vi "Average tau0.vi"(4 "filter changed?":bool, 6 "filter":bool, 8 "error in":errorcluster, 9 "# of shots":i32, 10 "extParam":T1={"Tau"=nan, "Tau0cor"=nan, "ext"=nan, "extCorr"=nan, "stdevTau"=nan, "eTau"=nan, "taucorr"=nan, "Tau0"=nan, "max"=nan}, 11 "CRDS Cell in":refnum<class "CRDS Cell.lvclass">) -> (0 "error out":errorcluster, 3 "CRDS Cell out":refnum<class "CRDS Cell.lvclass">)   [LabVIEW 2014, in "CRDS Lib.lvlib" / "CRDS Cell.lvclass"]
doc: "Average taus recorded on filter to give a mean tau0. The values tau0 and tau0cor will be averaged over the number of times this vi is called or the value of <b># of shots</b>, whichever is smaller.\n\nOnly accessors can throw errors here."
uses:
  CRDS Cell.lvclass
  extParam Ctl.ctl
  CRDS Cell.lvclass/CRDS Cell.ctl
  Data/Cell/CRDS Cell Data.lvclass/CRDS Cell Data.ctl
  <vilib>/Analysis/baseanly.llb/Mean (DBL).vi
  Read Data.vi
  Data/Cell/Write extParam.vi
  Write Data.vi
  Write corr tau0.vi
  Write tau_0.vi
  Data/Cell/CRDS Cell Data.lvclass
  <vilib>/Analysis/NI_AALBase.lvlib
  CRDS Lib.lvlib
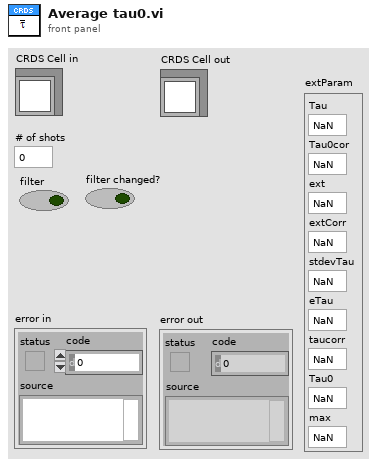
[diagram p1: front panel]
types:
  T1 = typedef "CRDS Lib.lvlib/extParam Ctl.ctl" = cluster{"Tau":sgl, "Tau0cor":sgl, "ext":sgl, "extCorr":sgl, "stdevTau":sgl, "eTau":sgl, "taucorr":sgl, "Tau0":sgl, "max":sgl}
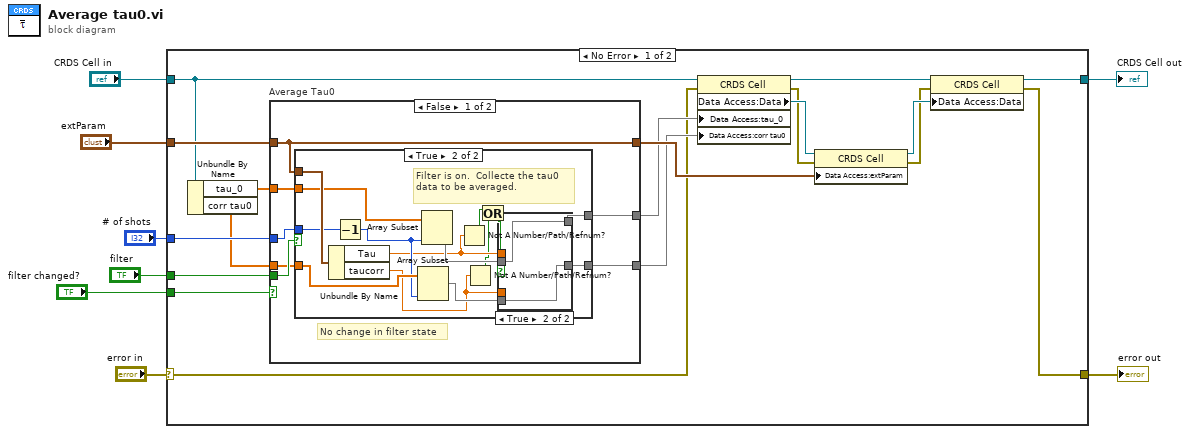
[diagram p0: block diagram]
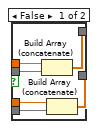
[diagram p3: hidden frame]
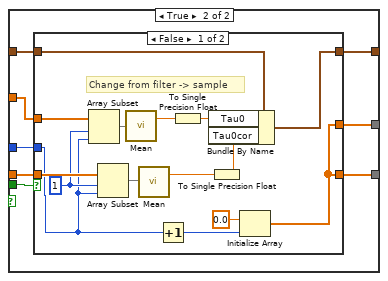
[diagram p4: hidden frame]
diagram:
  n1 = case shown="No Error" "error in" {
    selector: "error in" -> [w13 w85]
    tunnel: [w10 w85] -> w7
    tunnel: [w19 w84] -> w5
    tunnel: "CRDS Cell in" -> [w18 w84]
    tunnel: "extParam" -> [w26 _]
    tunnel: "# of shots" -> [w25 _]
    tunnel: "filter" -> [w24 _]
    tunnel: "filter changed?" -> [w9 _]
    frame No Error {
      n2 = Unbundle By Name(w18) -> ("tau_0"=w17:dbl[], "corr tau0"=w16:dbl[])
      n3 = case "Average Tau0" shown="False" w9 {
        tunnel: w24 -> [w30 w65]
        tunnel: w26 -> [w33 w64]
        tunnel: [w33 w63] -> w22
        tunnel: w17 -> [w32 w62]
        tunnel: [w31 w61] -> w14
        tunnel: w16 -> [w29 w60]
        tunnel: [w28 w59] -> w15
        tunnel: w25 -> [w27 w58]
        frame False {
          # "No change in filter state"
          n4 = case shown="True" w30 {
            tunnel: w33 -> [_ w49]
            tunnel: w32 -> [w35 w46]
            tunnel: [w35 w48] -> w31
            tunnel: w29 -> [w34 w44]
            tunnel: [w34 w41] -> w28
            tunnel: w27 -> [_ w47]
            frame False {
              # "On sample."
            }
            frame True {
              # "Filter is on.  Collecte the tau0  data to be averaged."
              n5 = Unbundle By Name(w49) -> ("Tau"=w40:sgl, "taucorr"=w39:sgl)
              n6 = Decrement(x=w47) -> (x-1=w43:i32)
              n7 = Array Subset(array=w44, length=w43) -> (w42:dbl[])  [unwired: 1 in]
              n8 = Array Subset(array=w46, length=w43) -> (w45:dbl[])  [unwired: 1 in]
              n9 = Not A Number/Path/Refnum?(number/path/refnum=w40) -> (NaN/Path/Refnum?=w38:bool)
              n10 = Not A Number/Path/Refnum?(number/path/refnum=w39) -> (NaN/Path/Refnum?=w37:bool)
              n11 = Or(x=w38, y=w37) -> (x .or. y?=w36:bool)
              n12 = case shown="True" w36 {
                tunnel: w40 -> [w55 _]
                tunnel: [w54 w57] -> w48
                tunnel: w45 -> [w53 w57]
                tunnel: w42 -> [w52 w56]
                tunnel: w39 -> [w51 _]
                tunnel: [w50 w56] -> w41
                frame False {
                  n13 = Build Array (concatenate)(w55, w53) -> (w54:dbl[])
                  n14 = Build Array (concatenate)(w51, w52) -> (w50:dbl[])
                }
                frame True {
                }
              }
            }
          }
        }
        frame True {
          n15 = case shown="False" w65 {
            tunnel: w64 -> [w80 w83]
            tunnel: [w79 w83] -> w63
            tunnel: w62 -> [w71 w82]
            tunnel: [w73 w82] -> w61
            tunnel: w60 -> [w70 w81]
            tunnel: [w73 w81] -> w59
            tunnel: w58 -> [w68 _]
            frame False {
              w69 = 1 ("index")
              # "Change from filter -> sample"
              n16 = Array Subset(array=w71, index=w69, length=w68) -> (w67:dbl[])
              n17 = Array Subset(array=w70, index=w69, length=w68) -> (w66:dbl[])
              n18 = call-poly <vilib>:"Mean.vi"("X"=w67) -> ("mean"=w78:dbl)  [unwired: 1 out]
              n19 = call-poly <vilib>:"Mean.vi"("X"=w66) -> ("mean"=w76:dbl)  [unwired: 1 out]
              n20 = Increment(x=w68) -> (x+1=w72:i32)
              n21 = To Single Precision Float(number=w78) -> (single precision float=w77:sgl)
              n22 = To Single Precision Float(number=w76) -> (single precision float=w75:sgl)
              n23 = Bundle By Name(cluster=w80, "Tau0"=w77, "Tau0cor"=w75) -> (w79:T1)
              n24 = Initialize Array(0.0, w72) -> (w73:dbl[])
            }
            frame True {
              # "Change from sample -> filter. Do nothing, the matrices have already been zeroed."
            }
          }
        }
      }
      n25 = property class="CRDS Cell"(reference=w18, error in=w13, "Data Access:tau_0"=w14, "Data Access:corr tau0"=w15) -> (reference out=w21:refnum<class "CRDS Cell.lvclass">, error out=w12:errorcluster, "Data Access:Data"=w23:refnum<class "CRDS Cell Data.lvclass">)
      n26 = property class="CRDS Cell"(reference=w23, error in=w12, "Data Access:extParam"=w22) -> (reference out=w20:refnum<class "CRDS Cell Data.lvclass">, error out=w11:errorcluster)
      n27 = property class="CRDS Cell"(reference=w21, error in=w11, "Data Access:Data"=w20) -> (reference out=w19:refnum<class "CRDS Cell.lvclass">, error out=w10:errorcluster)
    }
    frame Error {
    }
  }
  "error out" <- w7
  "CRDS Cell out" <- w5
